vi "Logger_Initialize.vi"(8 "error in (no error)":errorcluster caption="错误输入（无错误）", 9 "LoggerName":string="软件名称", 10 "LoggerSavePath":path, 11 "LoggerSaveTime":T1) -> (0 "错误输出":errorcluster)   [LabVIEW 2019, in "Logger.lvclass"]
uses:
  <userlib>/Logger/Logger.lvclass
  <userlib>/Logger/Ctls/LoggerSaveTime.ctl
  <userlib>/Logger/SubVIs/Logger_Core.vi
panel:
  # "...\\LoggerSavePath\\datepath\\\nLoggerName\\LoggerKind-dataname.csv"
  # "日志文件保存的文件夹基路径"
  # "日志文件保存的文件夹"
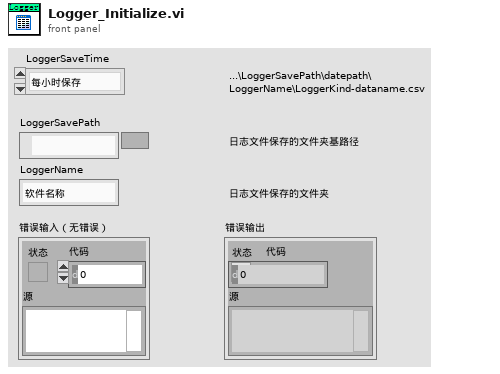
[diagram p1: front panel]
types:
  T1 = typedef "Logger.lvclass/LoggerSaveTime.ctl" = enum16{"每小时保存", "每天保存", "每周保存", "每月保存"}
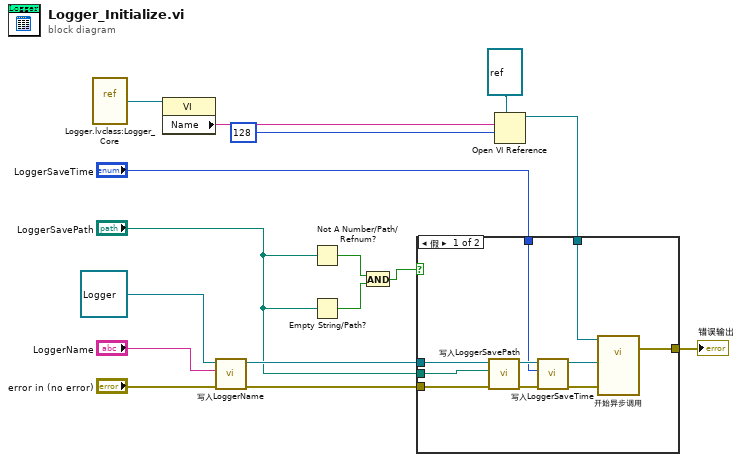
[diagram p0: block diagram]
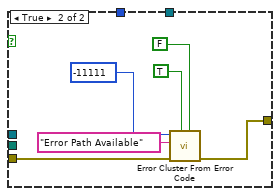
[diagram p2: hidden frame]
diagram:
  n1 = vi-ref "Logger.lvclass:Logger_Core.vi"() -> (w13:refnum<vi>)
  n2 = property class="VI"(reference=w13) -> ("Name"=w12:string)  [unwired: 1 in, 2 out]
  n3 = call "写入LoggerName.vi"("error in (no error)"="error in (no error)", "LoggerName"="LoggerName", "Logger输入"=refnum<class "Logger.lvclass"> refnum ("Logger.lvclass")) -> ("error out"=w2:errorcluster, "Logger输出"=w16:refnum<class "Logger.lvclass">)  [unwired: 7 in]
  n4 = Not A Number/Path/Refnum?(number/path/refnum="LoggerSavePath") -> (NaN/Path/Refnum?=w5:bool)
  n5 = Empty String/Path?(string/path="LoggerSavePath") -> (empty?=w4:bool)
  n6 = And(x=w5, y=w4) -> (x .and. y?=w3:bool)
  n7 = Open VI Reference(type specifier VI Refnum (for type only)=refnum<vi> refnum ("类型说明符VI引用句柄（仅用于类型）"), vi path=w12, options=128 ("选项")) -> (vi reference=w7:refnum<vi>)  [unwired: 3 in, 1 out]
  n8 = case shown="假" w3 {
    tunnel: w16 -> [w26 _]
    tunnel: w2 -> [w25 w32]
    tunnel: [w22 w29] -> w9
    tunnel: "LoggerSaveTime" -> [w21 _]
    tunnel: w7 -> [w20 _]
    tunnel: "LoggerSavePath" -> [w17 _]
    frame False {
      n9 = call "写入LoggerSavePath.vi"("error in (no error)"=w25, "LoggerSavePath"=w17, "Logger输入"=w26) -> ("error out"=w23:errorcluster, "Logger输出"=w24:refnum<class "Logger.lvclass">)  [unwired: 7 in]
      n10 = call "写入LoggerSaveTime.vi"("error in (no error)"=w23, "LoggerSaveTime"=w21, "Logger输入"=w24) -> ("error out"=w18:errorcluster, "Logger输出"=w19:refnum<class "Logger.lvclass">)  [unwired: 7 in]
      n11 = call-by-ref "开始异步调用"(reference=w20, "error in (no error)"=w18, "Logger 输入"=w19) -> (error out=w22:errorcluster)  [unwired: 9 in, 3 out]
    }
    frame True {
      n12 = call <vilib>:"Error Cluster From Error Code.vi"("is warning? (False)"=FALSE, "show call chain? (False)"=TRUE ("is warning? (False)"), "error in (no error)"=w32, "error message (\"\")"="Error Path Available" ("error message (\"\")"), "error code (0)"=-11111) -> ("error out"=w29:errorcluster)  [unwired: 4 in]
    }
  }
  "错误输出" <- w9
